vi "Joypad Loop.vi"() -> ()   [LabVIEW 2011]
doc: "This vi connects to a Joystick via Microsoft's Human Interface Devices and passes the necessary controls to the \"Remote\" variables \nSee Block Diagram:\n1. Quarry about available joystick\n2. Search for the joystick with the specified device\n3. If no match is found, then pass an error, then try and initialize the device\n4. Use a timed wile loop to save recourse, just looping and poling the joystick data is capable of high loop speeds\n5. Get Joystick sensor data\n6. Set the Trigger enable condition and pass along the XY data\n7. Normalize the values and use a running average to smooth out the control\n8. Apply expo weight for less sensitive control and zero out dead stick offset \n9. Set XY data\n10. XY plot is data binding to network variable for the XY plot on HUD from the Remote tab\n11. Use a stop button titled \"stop?\" so that the LabVIEW script can stop the vi\n12. Close the Joystick connection\n-Ruffin White\n-Kyle Green"
uses:
  <vilib>/Platform/TimedLoop/XDataNode/timing_clust.ctl
  <vilib>/Platform/TimedLoop/XDataNode/nitl_modes.ctl
  <vilib>/Platform/TimedLoop/XDataNode/wakeup.ctl
  <vilib>/Utility/inputDevices.llb/closeJoystick.vi
  <vilib>/Utility/inputDevices.llb/joystickAcquire.vi
  <vilib>/Platform/TimedLoop/XDataNode/XDataNode.xnode
  <vilib>/Platform/TimedLoop/XDataNode/XDNodeRunTimeDep.lvlib
panel:
  in  "Expo %":i32(slide)=1 scale=0.0..100.0
  out "button 3":bool
  out "x .and. y?":bool
  out "Y":dbl
  out "X":dbl
  out "X and Y":cluster{"X":dbl, "Y":dbl}
  out "Listed Devices":T1(array[cluster])
  out "Analog Stick":cluster{dbl, dbl}[](graph)
  out "error out":errorcluster
  in  "stop?":bool
  in  "Device Name":string="Controller (XBOX 360 For Windows)" caption="Give the exact \"divice name\" string of the joypad you would like to use."
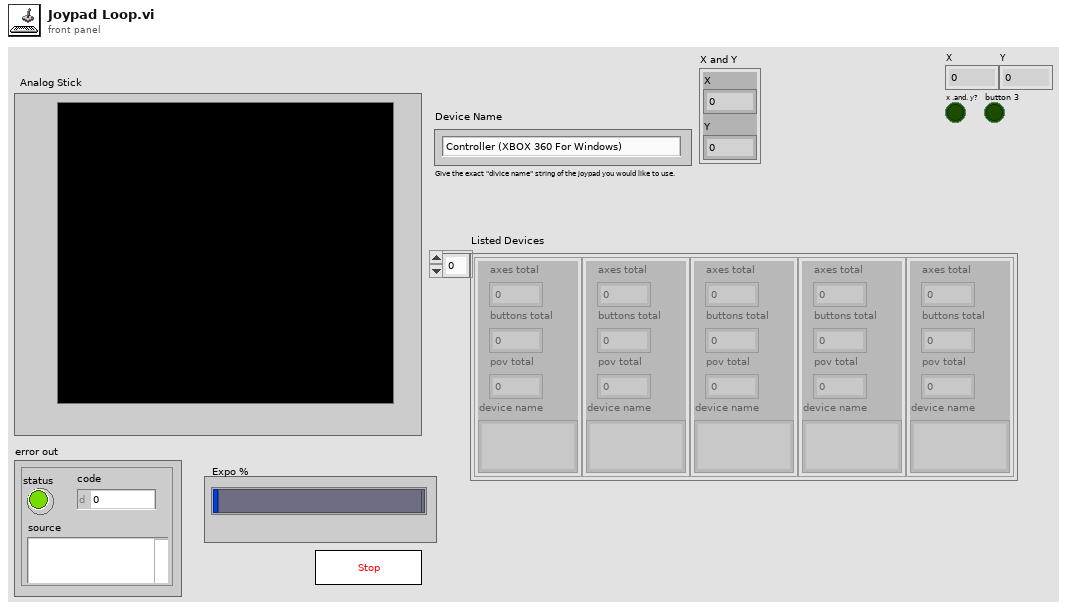
[diagram p1: front panel]
types:
  T1 = cluster{"axes total":u32, "buttons total":u32, "pov total":u32, "device name":string}[]
  T2 = typedef "XDNodeRunTimeDep.lvlib/timing_clust.ctl" = cluster{"Expected End [f-1]":u64, "Actual End [f-1]":u64, "Finished Late? [f-1]":bool, "Expected End [i-1]":u64, "Actual End [i-1]":u64, "Finished Late? [i-1]":bool, "Expected Start [i]":u64, "Actual Start [i]":u64, "Expected Start [f]":u64, "Actual Start [f]":u64, "Source Name":string, "Structure Name":string, "Period":i64, "Deadline":i64, "Offset":i64, "Start":i64, "Priority":i32, "Timeout":i32, "Mode":T3, "Wakeup Reason":T4, "Error":errorcluster, "Source Type":string, "Secondary Source Type":string, "Global End Time":u64, "Global Start Time":u64, "Frame Duration":u64, "Iteration Duration":u64, "Assigned CPU":i32, "I/O Scan Engine Mode":u32}
  T3 = typedef "XDNodeRunTimeDep.lvlib/nitl_modes.ctl" = enum32{"No Change", "Process missed periods, maintain original phase", "Discard missed periods, maintain original phase", "Process missed periods, ignore original phase", "Discard missed periods, ignore original phase"}
  T4 = typedef "XDNodeRunTimeDep.lvlib/wakeup.ctl" = enum32{"Normal", "Aborted", "Asynchronous wakeup", "Timing source error", "Timed loop error", "Timeout"}
  T5 = cluster{"X axis":i32, "Y axis":i32, "Z axis":i32, "X axis rotation":i32, "Y axis rotation":i32, "Z axis rotation":i32, "U axis":i32, "V axis":i32}
  T6 = cluster{"button 1":bool, "button 2":bool, "button 3":bool, "button 4":bool, "button 5":bool, "button 6":bool, "button 7":bool, "button 8":bool, "button 9":bool, "button 10":bool, "button 11":bool, "button 12":bool, "button 13":bool, "button 14":bool, "button 15":bool, "button 16":bool, "button 17":bool, "button 18":bool, "button 19":bool, "button 20":bool, "button 21":bool, "button 22":bool, "button 23":bool, "button 24":bool, "button 25":bool, "button 26":bool, "button 27":bool, "button 28":bool, "button 29":bool, "button 30":bool, "button 31":bool, "button 32":bool}
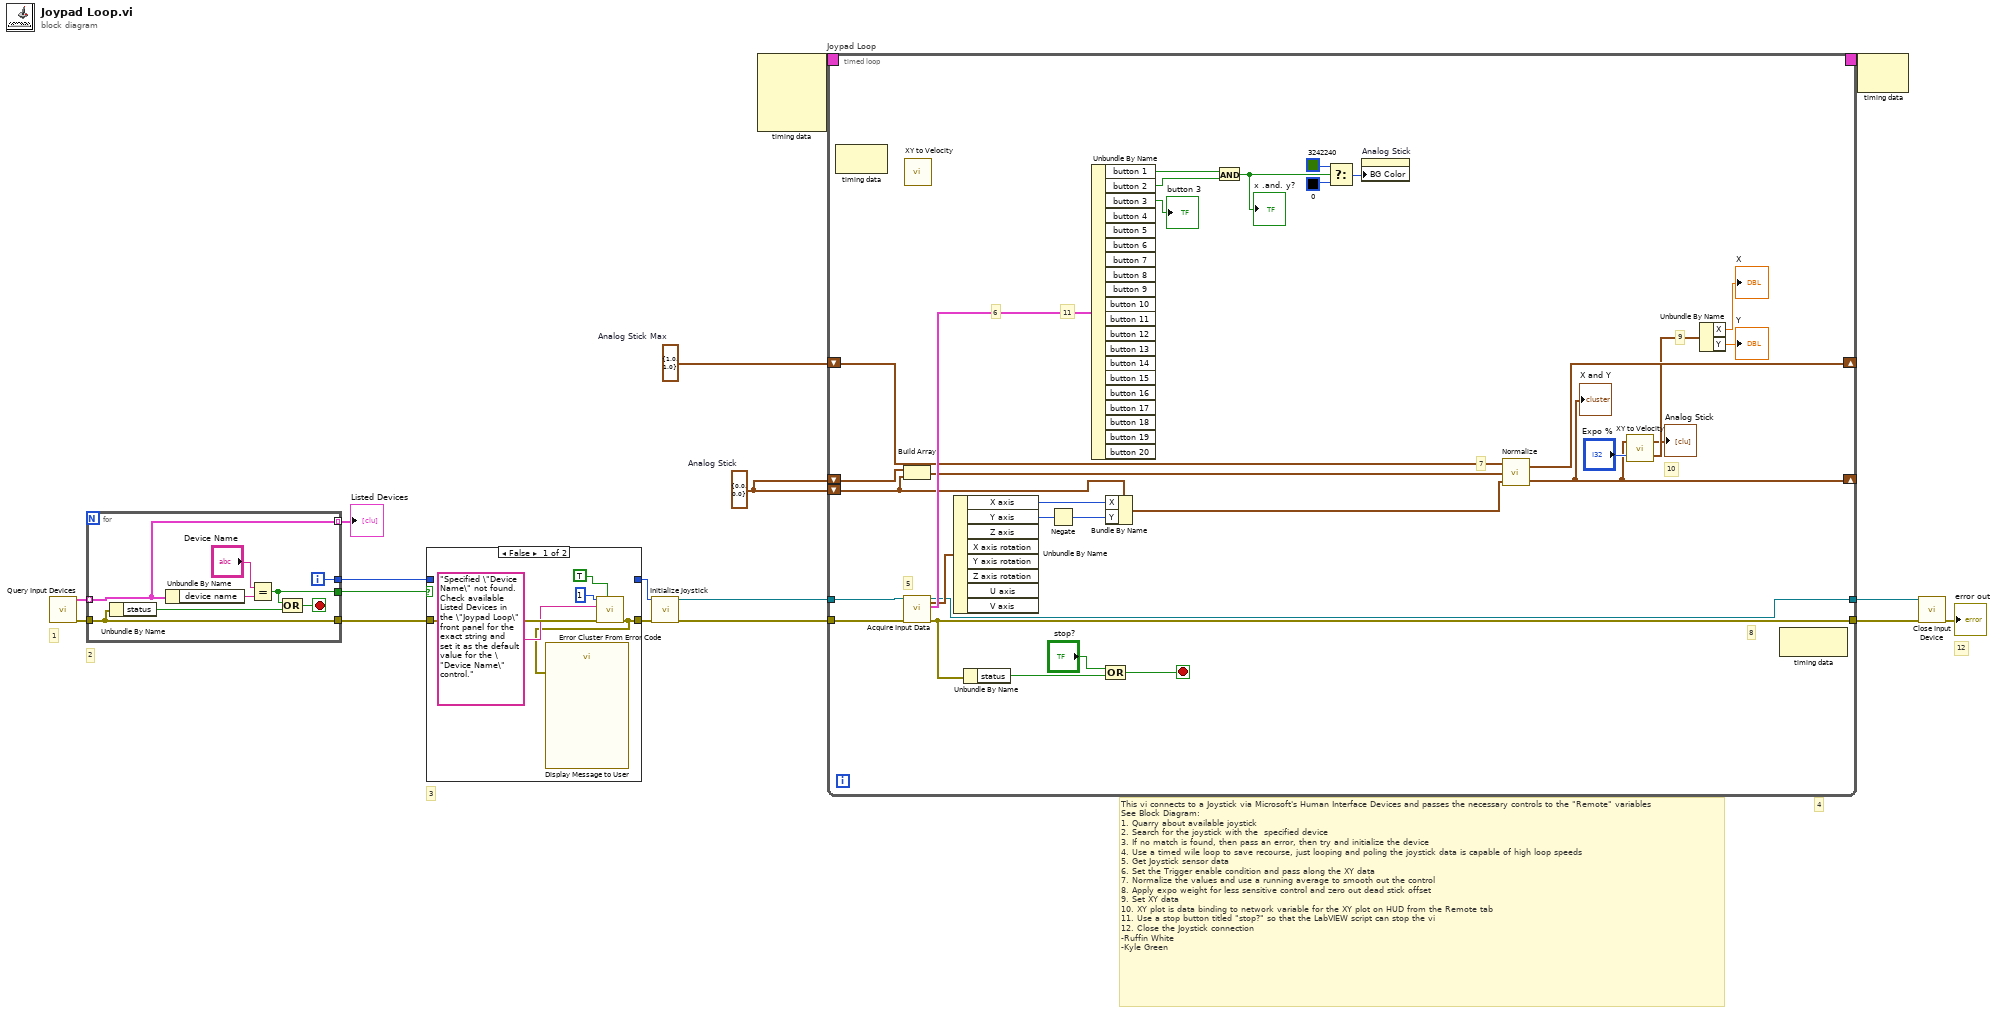
[diagram p0: block diagram]
diagram:
  w4 = cluster{"X":dbl, "Y":dbl} {"X"=1.0, "Y"=1.0}  # Analog Stick Max
  w2 = cluster{"X":dbl, "Y":dbl} {"X"=0.0, "Y"=0.0}  # Analog Stick
  # "This vi connects to a Joystick via Microsoft's Human Interface Devices and passes the necessary controls to the \"Remote\" variables   \nSee Block Diagram:\n1.\tQuarry about available joystick\n2.\tSearch for the joystick with the  specified device\n3.\tIf no match is found, then pass an error, then try and initialize the device\n4.\tUse a timed wile loop to save recourse, just looping and poling the joystick data is capable of high loop speeds\n5.\tGet Joystick sensor data\n6.\tSet the Trigger enable condition and pass along the XY data\n7.\tNormalize the values and use a running average to smooth out the control\n8.\tApply expo weight for less sensitive control and zero out dead stick offset \n9.\tSet XY data\n10.\tXY plot is data binding to network variable for the XY plot on HUD from the Remote tab\n11.\tUse a stop button titled \"stop?\" so that the LabVIEW script can stop the vi\n12.\tClose the Joystick connection\n-Ruffin White\n-Kyle Green"
  # "12"
  # "4"
  # "3"
  # "2"
  # "1"
  n1 = call <vilib>:"Query Input Devices.vi"() -> ("error out"=w10:errorcluster, "joystick info"=w13:T1)  [unwired: 8 in, 2 out]
  n2 = for {
    tunnel: w13 -> [w18] mode=indexing
    tunnel: [w23] -> w12
    tunnel: [w20] -> w11
    tunnel: w10 -> [w21]
    tunnel: [w21] -> w9
    tunnel: [w18] -> w8 mode=indexing
    i -> [w23]
    stop <- w22 stop-if-true
    n3 = Unbundle By Name(w21) -> ("status"=w19:bool)
    n4 = Unbundle By Name(w18) -> ("device name"=w24:string)
    n5 = Equal?(x="Device Name", y=w24) -> (x = y?=w20:bool)
    n6 = Compound Arithmetic op=OR(w20, w19) -> (w22:bool)
  }
  "Listed Devices" <- w8
  n7 = case shown="False" w11 {
    tunnel: w12 -> [_ w32]
    tunnel: [_ w32] -> w7
    tunnel: w9 -> [w30 w31]
    tunnel: [w26 w31] -> w1
    frame False {
      n8 = call <vilib>:"Error Cluster From Error Code.vi"("show call chain? (False)"=TRUE, "error in (no error)"=w30, "error message (\"\")"="Specified \"Device Name\" not found. Check available Listed Devices in the \"Joypad Loop\" front panel for the exact string and set it as the default value for the \"Device Name\" control." ("error message (\"\")"), "error code (0)"=1) -> ("error out"=w26:errorcluster)  [unwired: 5 in]
      n9 = call "Display Message to User"("error in (no error)"=w26) -> ()  [unwired: 9 in, 2 out]
    }
    frame True {
    }
  }
  n10 = call <vilib>:"Initialize Joystick.vi"("error in (no error)"=w1, "device index"=w7) -> ("error out"=w14:errorcluster, "device ID"=w17:refnum<k1>)  [unwired: 8 in]
  n11 = node-c288() -> (w6:T2)  [unwired: 4 in]
  n12 = timed-loop "Joypad Loop" {
    tunnel: w17 -> [w62]
    tunnel: [w55] -> w15
    tunnel: w14 -> [w58]
    shift-right: [w35] -> _
    shift-left: w2 -> [w50]
    timing: w6 -> [_]
    timing-out: [_] -> w5
    shift-right: [w51] -> _
    shift-left: w4 -> [w48]
    shift-left: w2 -> [w47]
    tunnel: [w45] -> w3
    stop <- w54 stop-if-true
    # "7"
    # "11"
    # "10"
    # "9"
    # "8"
    # "6"
    # "5"
    n13 = node-c288() -> ()  [unwired: 1 in, 1 out]
    n14 = Build Array(w50, w47) -> (w49:cluster{"X":dbl, "Y":dbl}[])
    n15 = call-poly <vilib>:"Acquire Input Data.vi"("device ID"=w62, "error in (no error)"=w58) -> ("device ID"=w45:refnum<k1>, "axis info"=w59:T5, "button info"=w63:T6, "error out"=w55:errorcluster)  [unwired: 13 in, 1 out]
    n16 = call "XY to Velocity.vi"() -> ()  [unwired: 2 in, 2 out]
    n17 = Unbundle By Name(w59) -> ("X axis"=w44:i32, "Y axis"=w39:i32)  [unwired: 6 out]
    n18 = Unbundle By Name(w55) -> ("status"=w52:bool)
    n19 = Negate(x=w39) -> (-x=w38:i32)
    n20 = Unbundle By Name(w63) -> ("button 1"=w61:bool, "button 2"=w60:bool, "button 3"=→"button 3":bool)  [unwired: 17 out]
    n21 = Bundle By Name(cluster=w47, "X"=w44, "Y"=w38) -> (w46:cluster{"X":dbl, "Y":dbl})
    n22 = Compound Arithmetic op=OR("stop?", w52) -> (w54:bool)
    n23 = And(x=w61, y=w60) -> (x .and. y?=w40:bool)
    "x .and. y?" <- w40
    n24 = Select(t=u32 3242240, s=w40, f=u32 0) -> (s? t:f=w43:u32)
    n25 = property on="Analog Stick" class="XYGraph (strict)"("BG Color"=w43) -> ()  [unwired: 2 in, 2 out]
    n26 = call "Normalize.vi"("Analog Stick"=w46, "Past Analog Stick"=w49, "Analog Stick Max"=w48) -> ("Normalized Analog Stick Out"=w35:cluster{"X":dbl, "Y":dbl}, "Analog Stick Max Out"=w51:cluster{"X":dbl, "Y":dbl})
    "X and Y" <- w35
    n27 = call "XY to Velocity.vi"("Expo"="Expo %", "Nunchuk Analog Stick In"=w35) -> ("X and Y"=w34:cluster{"X":dbl, "Y":dbl}, "Nunchuk Analog Stick"=→"Analog Stick":cluster{dbl, dbl}[])
    n28 = Unbundle By Name(w34) -> ("X"=→"X":dbl, "Y"=→"Y":dbl)
    n29 = node-c288() -> ()  [unwired: 1 in, 1 out]
  }
  n30 = node-c288(w5) -> ()  [unwired: 1 out]
  n31 = call-poly <vilib>:"Close Input Device.vi"("error in (no error)"=w15, "device ID"=w3) -> ("error out"=→"error out":errorcluster)  [unwired: 8 in]
